vi "Daten zusammensammeln HovaCal.vi"(1 "KommLoopTimer":u32, 5 "Aktionen Daten abholen":T2, 7 "Aktion Unterbrechen":T1, 11 "error in (no error)":errorcluster caption="Fehler (Eingang, kein Fehler)") -> (4 "Anzeige aktualisieren":bool, 6 "Aktionen Daten abholen":T2, 8 "Aktion Unterbrechen out":T1, 10 "Zustand":string, 15 "error out":errorcluster caption="Fehler (Ausgang)")   [LabVIEW 2020, in "Linearisierung v2.lvlib"]
uses:
  Linearisierung v2.lvlib
  Daten abholen.ctl
  Gasteiler/Aktion unterbrechen.ctl
  Gasteiler/Aktion FGV Daten Abholung uebergebenctl.ctl
  Aktion FGV Stoerungen sammeln und auswerten.ctl
  Funktionstasten/Funktionstasten-Aktion.ctl
  Funktionstasten/Zustaende.ctl
  Seiten/FT-IR/Algebraic Modul/FGV Algebraic Aktionen.ctl
  Sprachverwaltung/FGV Aktion Tabelle zerlegen.ctl
  Seiten/FT-IR/FGV FT-IR Gasliste Aktionen.ctl
  Gasteiler/Aktionen FGV Gasteiler Daten.ctl
  Aktion Lin Daten aufarbeiten.ctl
  SpanEinstellungen/Aktion FGV GD Errors sammeln.ctl
  SpanEinstellungen/GD Info Cluster.ctl
  LIN ErrorCluster.ctl
  Funktionstasten/Funktionstasten.lvlib
  Allgemein/allgemeine Sub-VIs.lvlib
  Sprachverwaltung/Sprachverwaltung.lvlib
  Gasteiler/Gasteiler.lvlib
  Gasteiler/HovaCal/HovaCal.lvlib
  Gasteiler/HovaCal/Aktion_FGV_Betriebsdaten.ctl
  Gasteiler/HovaCal/Aktion_FGV_Kom.ctl
  Seiten/FT-IR/Algebraic Modul/Algebraic Modul.lvlib
  Seiten/FT-IR/FT-IR.lvlib
  Gasteiler/HovaCAL_Interface/Kommunikation/Kommunikation.lvlib
  Gasteiler/HovaCAL_Interface/HovaCAL_Interface.lvlib
  SpanEinstellungen/SpanEinstellungen.lvlib
  Gasteiler/HovaCAL_Interface/Helper/Helper.lvlib
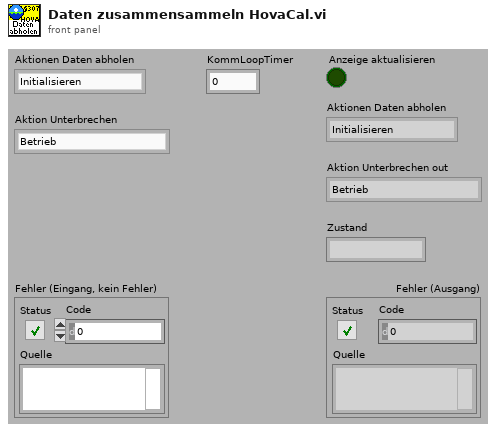
[diagram p1: front panel]
types:
  T1 = typedef "Linearisierung v2.lvlib/Gasteiler.lvlib/Aktion unterbrechen.ctl" = enum16{"Betrieb", "Unterbrechen", "Warten"}
  T2 = typedef "Linearisierung v2.lvlib/Daten abholen.ctl" = enum16{"Initialisieren", "Punkt aufschalten", "Warten", "Daten abholen", "Fertig", "Beenden", "Spülen", "Abbrechen"}
  T3 = typedef "Linearisierung v2.lvlib/Gasteiler.lvlib/Aktion FGV Daten Abholung uebergebenctl.ctl" = enum16{"lesen", "schreiben", "Anzeigebit löschen", "Status hinzufügen"}
  T4 = typedef "Linearisierung v2.lvlib/Aktion FGV Stoerungen sammeln und auswerten.ctl" = enum16{"init", "lesen", "error", "prüfen", "reset error", "abbrechen", "fortsetzen", "neustart", "Bedientasten reset"}
  T5 = typedef "Funktionstasten.lvlib/Zustaende.ctl" = enum16{"Standby", "Pause", "Eco", "Messen", "Kalibrieren", "Spülen Filter", "Spülen Leitung", "Umgebungsluft", "0-Gas", "Cal-Gas", "CG zu PNS", "-------------", "Init 1", "Init 2", "Init 3", "Init 4", "Messen vorbereiten", "Messen durchführen", "Exit"}
  T6 = typedef "Funktionstasten.lvlib/Funktionstasten-Aktion.ctl" = enum16{"Initialisieren", "Zustand setzen", "Taste gedrückt", "Fehler speichern", "Lesen", "Manuell", "Remote", "Bitparallel", "Samplepoint", "Zeit Prüfen", "reset Umschalten"}
  T7 = typedef "Linearisierung v2.lvlib/Aktion Lin Daten aufarbeiten.ctl" = enum16{"lesen", "Protkolldaten", "speichern", "laden", "EPA auswerten", "Tabelle schreiben", "Lin auswerten", "Tab init", "Stufentabelle", "EPA aktiviert", "Nachbehandlung laden", "Tabelle löschen", "Istwerte löschen", "Zeile löschen", "Zeile einfügen", "LIN aktiviert", "LIN/EPA aktiv laden", "EGAK Tab", "LIN übernehmen", "Tab init ohne Stufen"}
  T8 = typedef "Linearisierung v2.lvlib/Gasteiler.lvlib/Aktionen FGV Gasteiler Daten.ctl" = enum16{"lesen", "Gasteiler Daten", "Seriellen Param.", "MB-Endwert", "laden", "speichern", "Anforderung", "TCP", "Aufzeichnung Start"}
  T9 = typedef "FT-IR.lvlib/FGV FT-IR Gasliste Aktionen.ctl" = enum16{"lesen", "Gasliste FT-IR", "Gasliste ausgelesen", "laden", "speichern", "löschen"}
  T10 = typedef "Sprachverwaltung.lvlib/FGV Aktion Tabelle zerlegen.ctl" = enum16{"laden", "vereinzeln", "speichern"}
  T11 = typedef "FT-IR.lvlib/Algebraic Modul.lvlib/FGV Algebraic Aktionen.ctl" = enum16{"lesen", "laden", "speichern", "berechnen", "schreiben"}
  T12 = typedef "Linearisierung v2.lvlib/Gasteiler.lvlib/HovaCal.lvlib/Aktion_FGV_Kom.ctl" = enum16{"Initialisieren", "Betriebsparameter", "Gase", "Vaporizer", "Dynamische Werte", "Beenden", "Com ändern", "Gase init"}
  T13 = typedef "Linearisierung v2.lvlib/Gasteiler.lvlib/HovaCal.lvlib/Aktion_FGV_Betriebsdaten.ctl" = enum16{"Lesen", "Sollwerte schreiben", "Sollwerte lesen", "Gase schreiben", "Gase lesen", "Dynamische Werte", "GaseRef", "Gase aendern"}
  T14 = typedef "Linearisierung v2.lvlib/SpanEinstellungen.lvlib/GD Info Cluster.ctl" = cluster{"Wobei":string, "Status":string, "Errors":T15, "Empfangsdaten":string[], "Zeitstempel":string}
  T15 = typedef "Linearisierung v2.lvlib/LIN ErrorCluster.ctl" = cluster{"Störung Kommunikation":bool, "Pressure carrier gas":bool, "Pressure diluted gas":bool, "Outlet Pressure":bool, "SNOX before SAIR":bool, "Störung Gasteiler":bool}
  T16 = typedef "Linearisierung v2.lvlib/SpanEinstellungen.lvlib/Aktion FGV GD Errors sammeln.ctl" = enum16{"lesen", "init", "GD Infos sammeln", "Kalibrierinfos sammeln", "Test Data", "GD Infos selektiv sammeln"}
  T17 = typedef "Linearisierung v2.lvlib/Gasteiler.lvlib/HovaCal.lvlib/Betriebsdaten.ctl" = cluster{"Gesamtdurchfluss":dbl, "Eingangskonzentration \nTrägergas":dbl, "Eingangskonzentration\nKomponente 1":dbl, "Eingangskonzentration \nKomponente 2":dbl, "Ausgangskonzentration \nKomponente 1 ":dbl, "Ausgangskonzentration\nKomponente 2":dbl, "l/min -> ml/min":bool, "N2 %->ppm":bool, "Komp1 ppm->%":bool, "Komp2ppm->%":bool, "Sollkomp1ppm->%":bool, "Sollkomp2ppm->%":bool}
  T18 = typedef "Linearisierung v2.lvlib/Lin-Polynom Daten.ctl" = cluster{"Messgerät":string, "Kalibrator (Gasteiler)":string, "Bearbeiter/in":string, "Komponente":string, "Zeitstempel":timestamp, "F_max gefordert (%)":sgl, "F_max in %":sgl, "F_max in ppm":sgl, "Vorschlag Ordnung":i32, "Polynom OK":bool, "Polynomkoeff.":dbl[], "Prüfgas Konzentration":dbl, "Pfad EPA":string, "Pfad_LIN":string, "Gasnummer:":u8, "Komponentenauswahl":T19, "Verdünnungsgas":T21, "Zeitdauer Stufe":T22, "Anzahl Stufen":T22, "F_max in % EPA":sgl, "F_max in ppm EPA":sgl, "F_max in % LIN":sgl, "F_max in ppm LIN":sgl, "Punkte umkehren":bool, "EPA Optionsfeld":T23, "Autolin Hovacal":T24, "Spanfactors":sgl[], "Kalibrierauswahl":T25, "Conditions:":T26, "Gasflaschen Nr.:":string, "Bottle Accuracy":dbl, "Konfig Gasflasche":T27, "Gasflasche":T28, "HovaCAL Flow AutoLin":T29, "MFC Output":T30, "Gas Ablaufdatum":timestamp, "Lin Modus":T31, "zusätzliche Zeitdauer Erster Punkt":sgl, "Offsets":sgl[]}
  T19 = typedef "Linearisierung v2.lvlib/KomponentenArray.ctl" = cluster{"Komponente:":T20, "Konzentration":dbl}[]
  T20 = typedef "Auswahlfeld.ctl" = u16
  T21 = typedef "Linearisierung v2.lvlib/Gasteiler.lvlib/Prüfgas in.ctl" = u16
  T22 = typedef "Zahlen-Eingabefeld.ctl" = sgl
  T23 = typedef "Linearisierung v2.lvlib/EPA Optionsfeld.ctl" = enum32{"Istwert", "Rohwert", "Linearisierter Wert"}
  T24 = typedef "Linearisierung v2.lvlib/Gasteiler.lvlib/HovaCal.lvlib/AutoLin Hovacal.ctl" = enum32{"Keine Auswahl", "Optionsauswahl 1", "Optionsauswahl 2"}
  T25 = typedef "Linearisierung v2.lvlib/Kalibrieroption.ctl" = u16
  T26 = typedef "Linearisierung v2.lvlib/Linearity verification 1065-307.lvlib/Condition.ctl" = u16
  T27 = typedef "System Einstellungen V2.lvlib/Konfig Gasflasche.ctl" = bool
  T28 = typedef "System Einstellungen V2.lvlib/Gasflasche Auswahl.ctl" = u16
  T29 = typedef "Linearisierung v2.lvlib/Gasteiler.lvlib/HovaCAL_Interface.lvlib/Controls.lvlib/Flow Einstellung.ctl" = cluster{"HovaCAL Flow Input Cluster":dbl}
  T30 = typedef "Linearisierung v2.lvlib/Gasteiler.lvlib/HovaCAL_Interface.lvlib/Controls.lvlib/Pump state.ctl" = cluster{"Run":bool}
  T31 = typedef "CalGas Aufschaltung.lvlib/Lin Modus.ctl" = u16
  T32 = typedef "String - Ausgabefeld.ctl" = string
  T33 = typedef "Linearisierung v2.lvlib/Gasteiler.lvlib/Stufen Tabelle.ctl" = string[][]
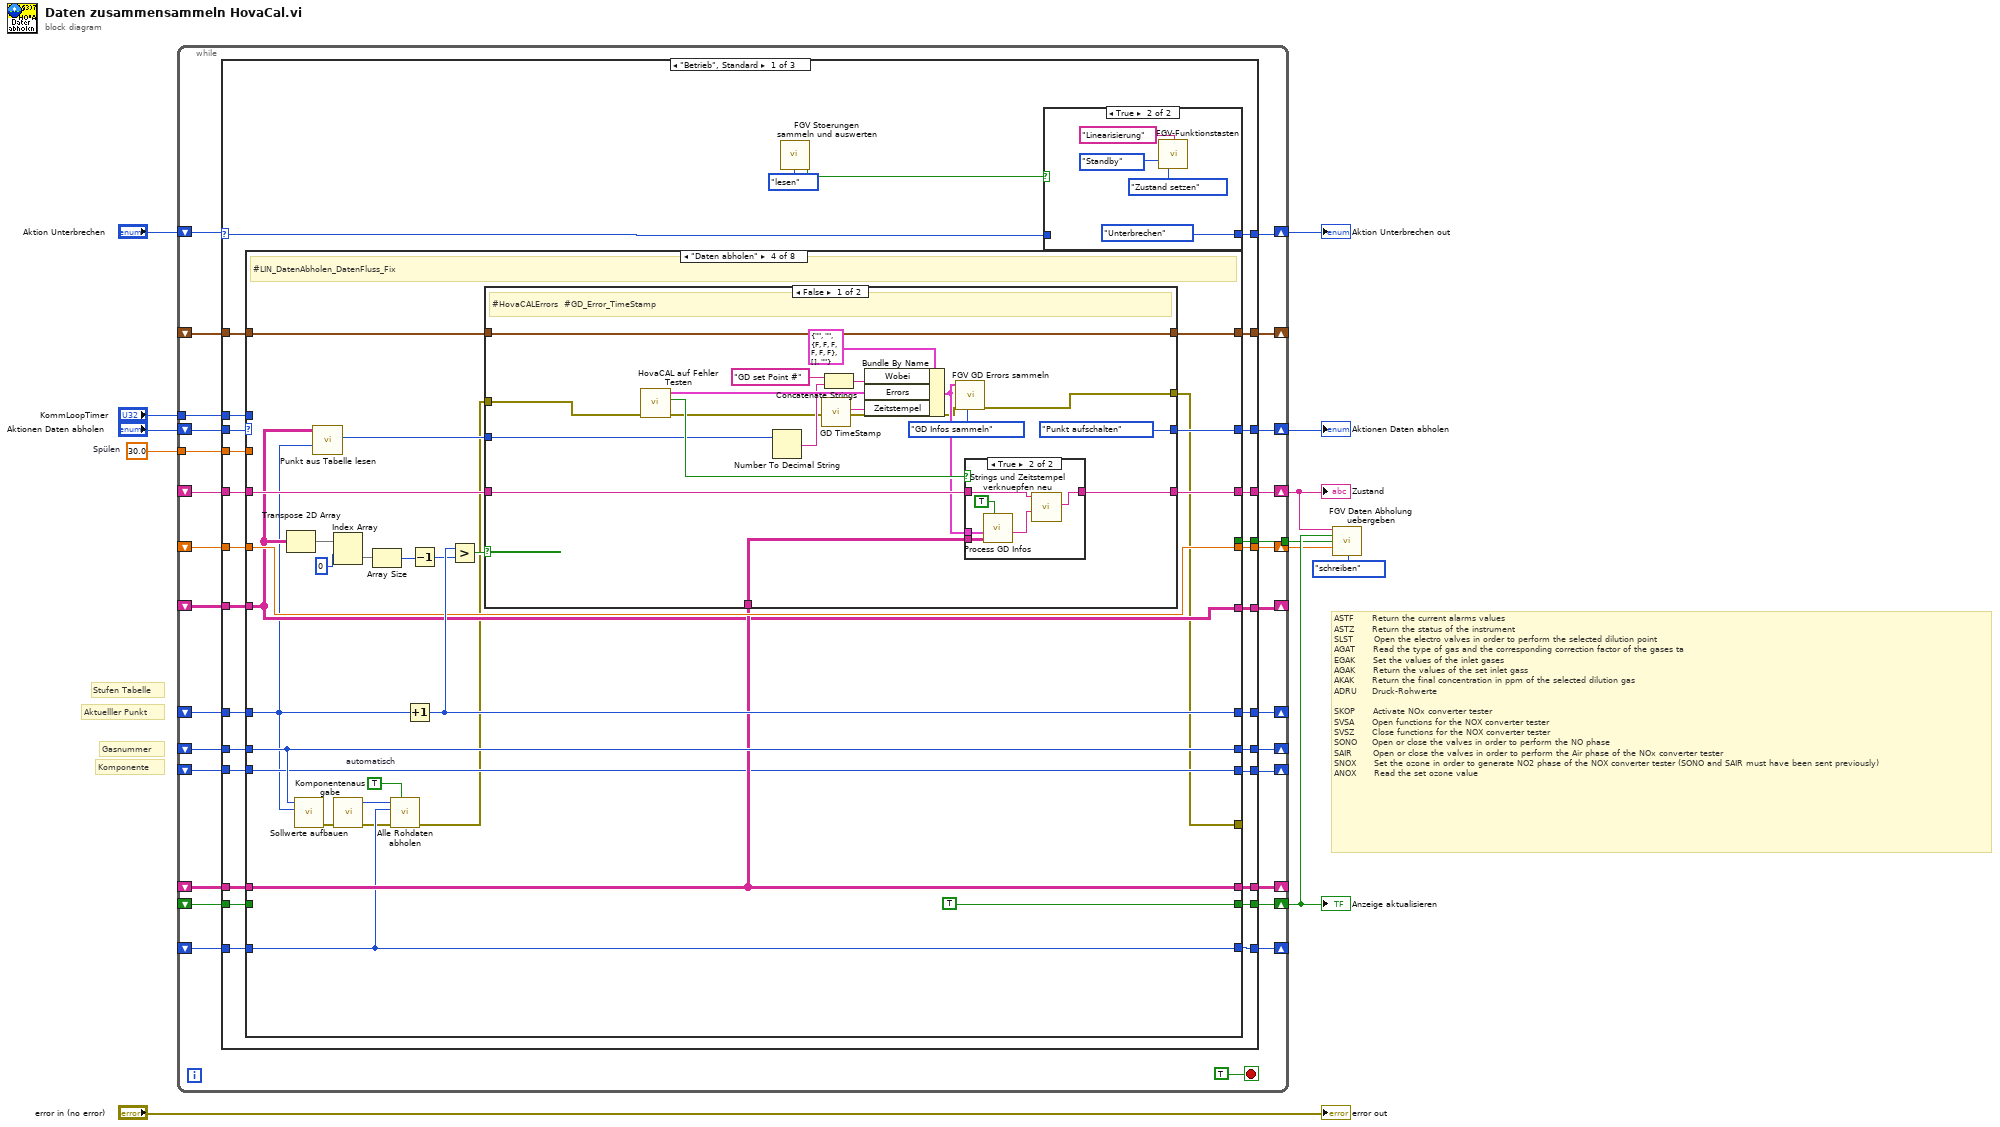
[diagram p0: block diagram]
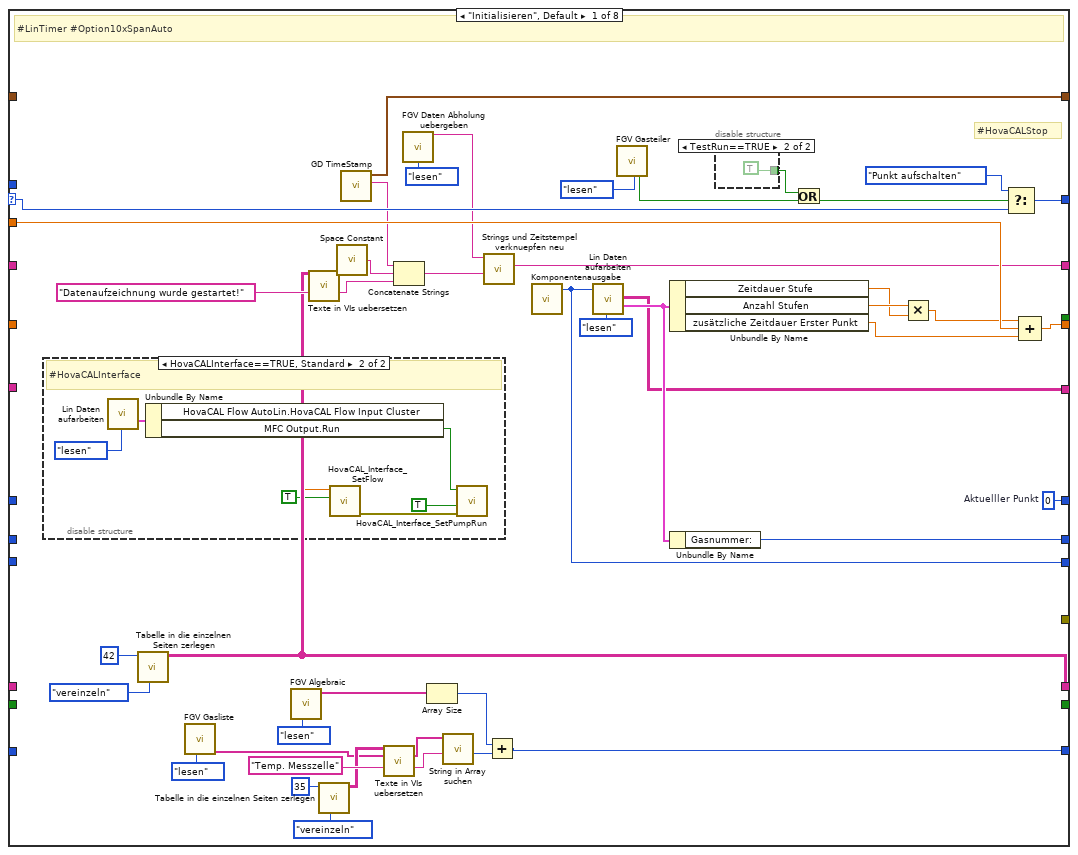
[diagram p3: hidden frame]
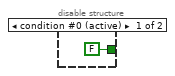
[diagram p4: hidden frame]
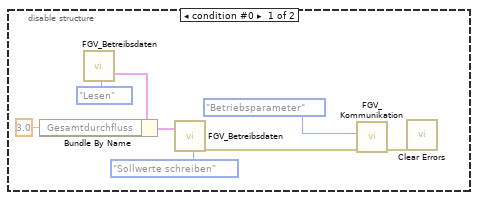
[diagram p5: hidden frame]
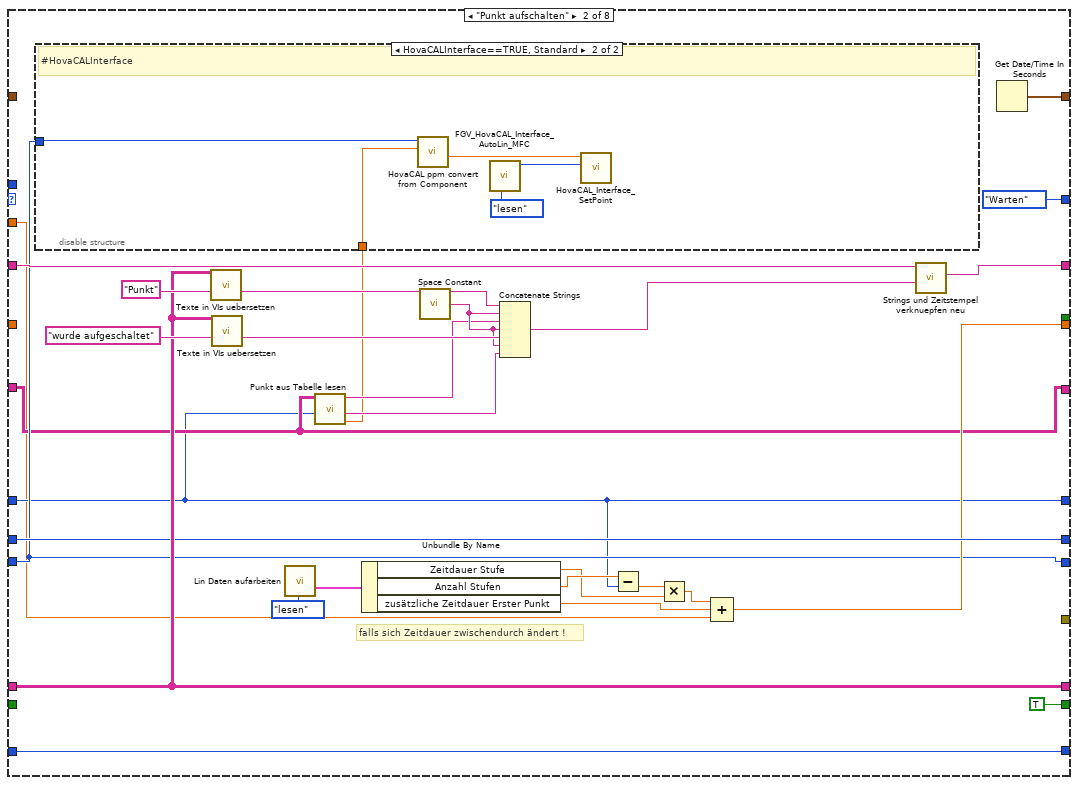
[diagram p6: hidden frame]
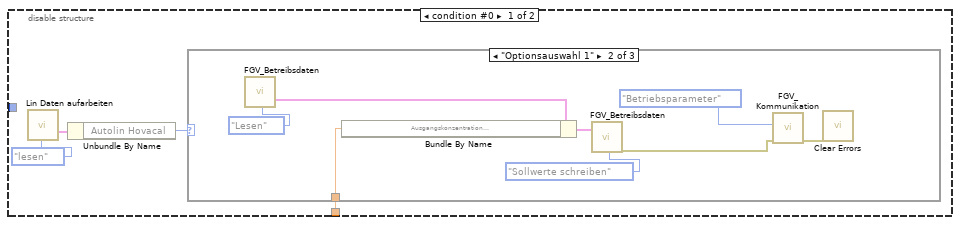
[diagram p7: hidden frame]
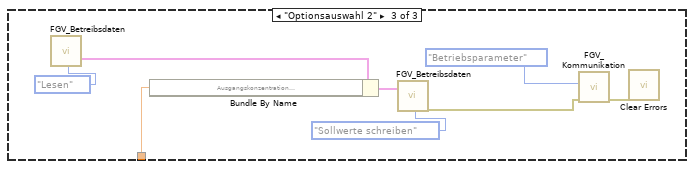
[diagram p9: hidden frame]
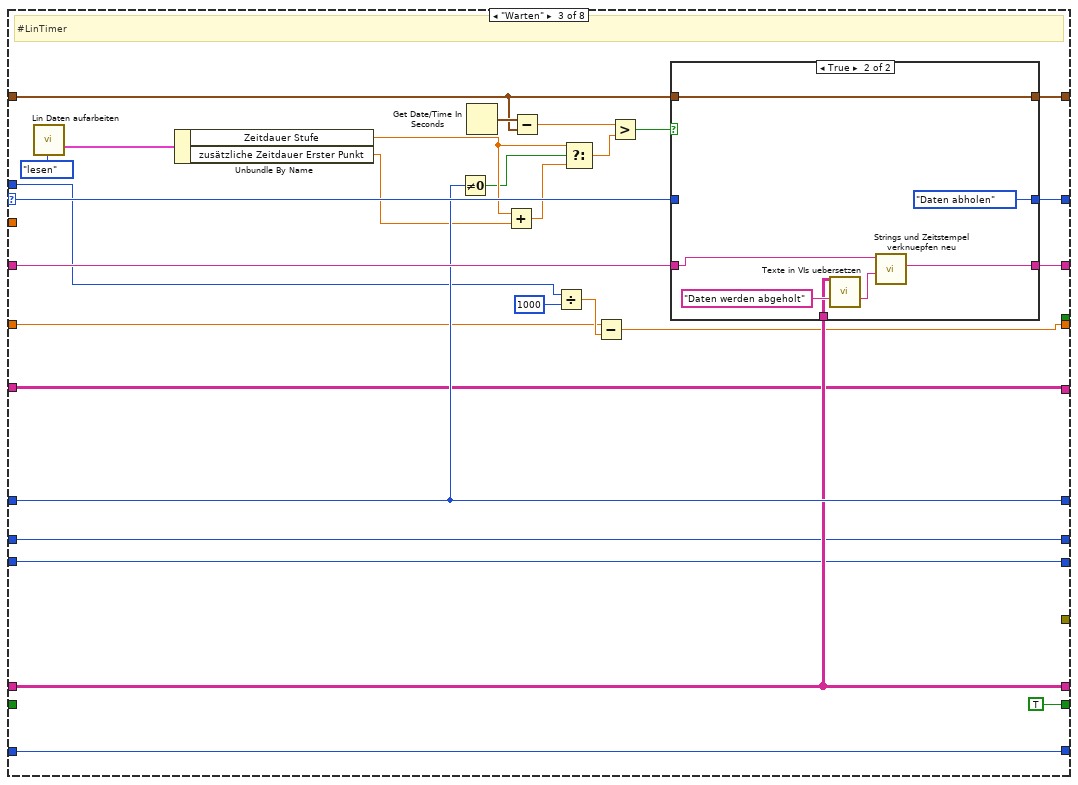
[diagram p10: hidden frame]
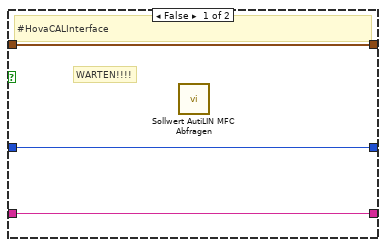
[diagram p11: hidden frame]
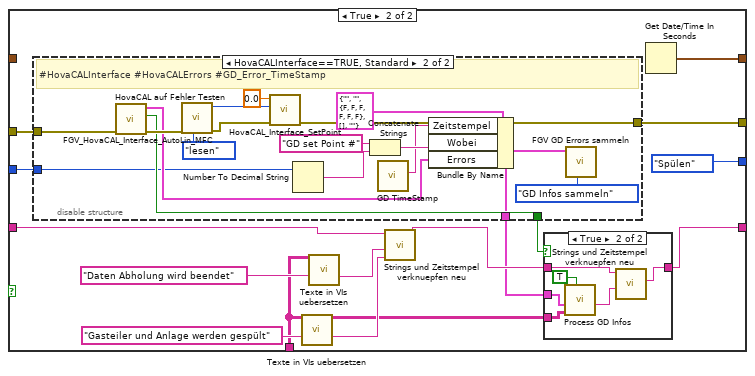
[diagram p13: hidden frame]
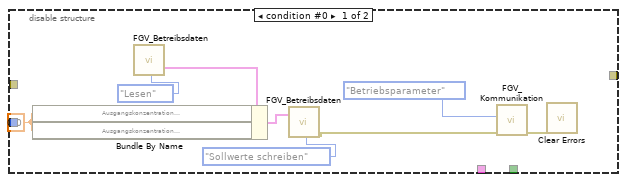
[diagram p15: hidden frame]
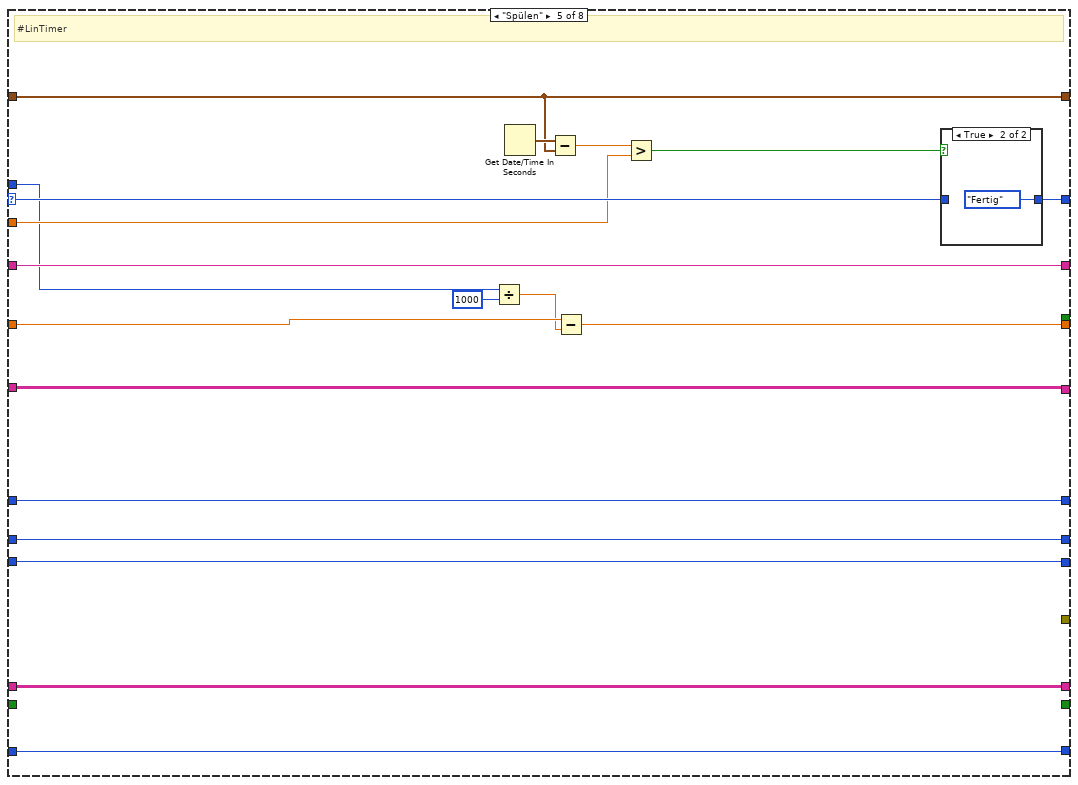
[diagram p16: hidden frame]
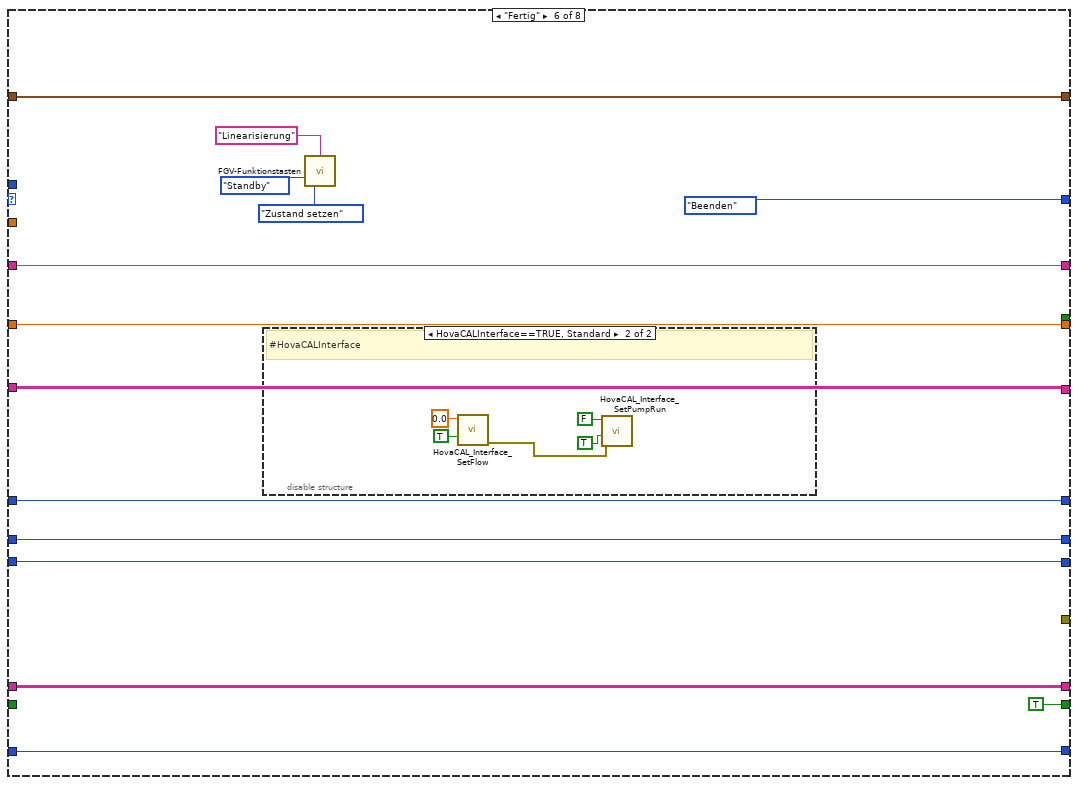
[diagram p18: hidden frame]
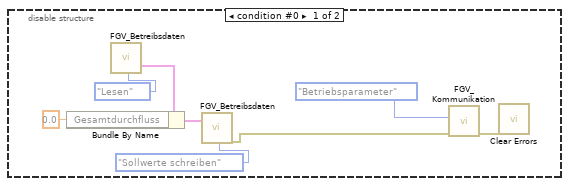
[diagram p19: hidden frame]
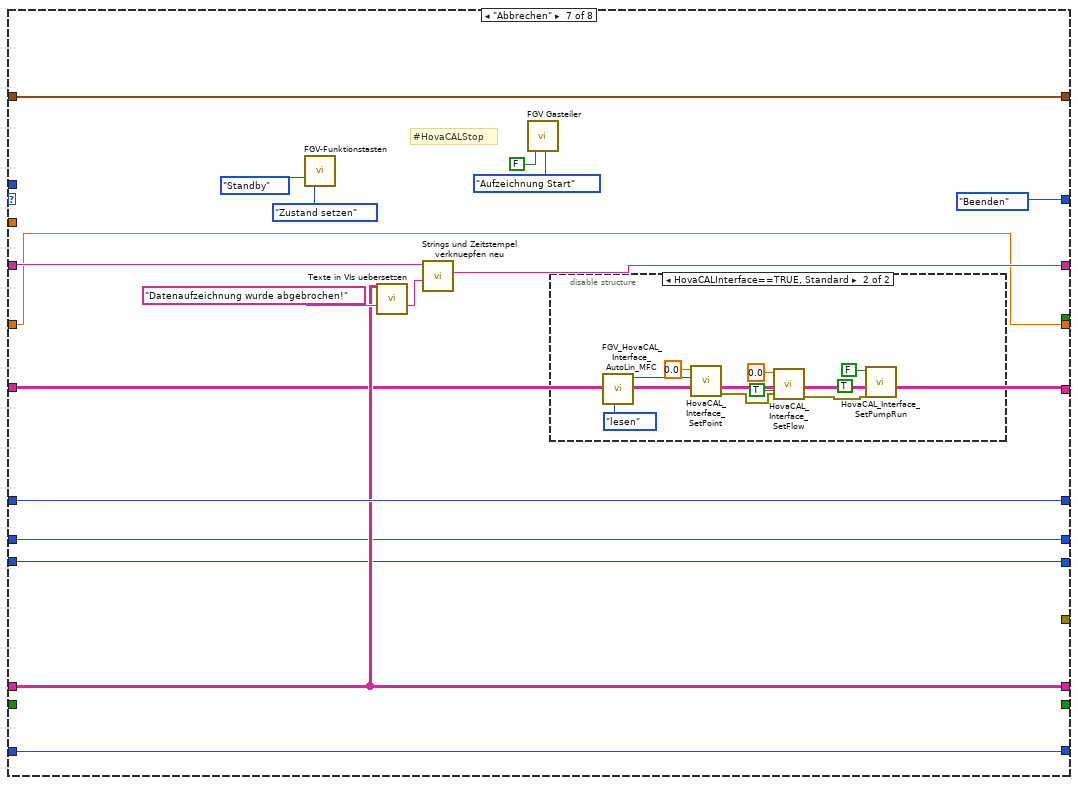
[diagram p20: hidden frame]
diagram:
  w5 = 30.0  # Spülen
  # "Komponente"
  # "Gasnummer"
  # "ASTF      Return the current alarms values\nASTZ      Return the status of the instrument \nSLST       Open the electro valves in order to perform the selected dilution point \nAGAT      Read the type of gas and the corresponding correction factor of the gases ta \nEGAK      Set the values of the inlet gases \nAGAK      Return the values of the set inlet gass \nAKAK      Return the final concentration in ppm of the selected dilution gas \nADRU     Druck-Rohwerte \n\nSKOP      Activate NOx converter tester \nSVSA      Open functions for the NOX converter tester \nSVSZ      Close functions for the NOX converter tester\nSONO     Open or close the valves in order to perform the NO phase\nSAIR       Open or close the valves in order to perform the Air phase of the NOx converter tester\nSNOX      Set the ozone in order to generate NO2 phase of the NOX converter tester (SONO and SAIR must have been sent previously)\nANOX      Read the set ozone value"
  # "Stufen Tabelle"
  # "Aktuelller Punkt"
  n1 = while {
    shift-right: [w38] -> _
    shift-left: _ -> [w39]
    shift-right: [w35] -> w10
    shift-left: _ -> [w34]
    shift-right: [w33] -> _
    shift-left: _ -> [w36]
    shift-right: [w30] -> _
    shift-left: _ -> [w31]
    shift-right: [w29] -> w9
    shift-left: _ -> [w28]
    shift-right: [w27] -> _
    shift-left: _ -> [w26]
    shift-right: [w37] -> w12
    shift-left: "Aktionen Daten abholen" -> [w40]
    tunnel: [w25] -> w8
    shift-right: [w24] -> _
    shift-left: _ -> [w23]
    shift-right: [w22] -> w6
    shift-left: _ -> [w21]
    tunnel: w5 -> [w20]
    tunnel: "KommLoopTimer" -> [w19]
    shift-right: [w17] -> w1
    shift-left: "Aktion Unterbrechen" -> [w18]
    shift-right: [w16] -> _
    shift-left: _ -> [w15]
    shift-right: [w14] -> _
    shift-left: _ -> [w13]
    stop <- TRUE stop-if-true
    n2 = case shown="\"Betrieb\", Standard" w18 {
      selector: w18 -> [w46 _ w460]
      tunnel: w40 -> [w69 w436 w454]
      tunnel: w39 -> [w68 w437 w470]
      tunnel: [w67 w437 w470] -> w38
      tunnel: [w66 w436 w458] -> w37
      tunnel: w36 -> [w65 w429 w467]
      tunnel: [w64 w432 w456] -> w35
      tunnel: w34 -> [w63 w433 w457]
      tunnel: [w62 w429 w467] -> w33
      tunnel: w31 -> [w61 w428 w455]
      tunnel: [w60 w428 w455] -> w30
      tunnel: [w59 w427 w469] -> w29
      tunnel: w28 -> [w58 w427 w469]
      tunnel: [w57 w426 w468] -> w27
      tunnel: w26 -> [w56 w426 w468]
      tunnel: [w55 _ _] -> w25
      tunnel: [w54 w430 w466] -> w24
      tunnel: w23 -> [w53 w430 w466]
      tunnel: [w52 w431 w465] -> w22
      tunnel: w21 -> [w51 w431 w465]
      tunnel: w20 -> [w50 _ _]
      tunnel: w19 -> [w49 _ _]
      tunnel: [w45 Aktion_unterbrechen."Warten" ("Aktion Unterbrechen") w459] -> w17
      tunnel: [w44 w425 w453] -> w16
      tunnel: w15 -> [w43 w425 w453]
      tunnel: [w42 w424 w452] -> w14
      tunnel: w13 -> [w41 w424 w452]
      frame "Betrieb", Default {
        n3 = case shown="\"Daten abholen\"" w69 {
          selector: w69 -> [w94 _ w209 _ w339 _ _ w421]
          tunnel: w68 -> [_ _ w210 w249 w341 w361 w391 w420]
          tunnel: [w75 w164 w211 w248 w341 w361 w391 w420] -> w67
          tunnel: [w97 Daten_abholen."Warten" ("Aktionen Daten abholen") w214 w254 w345 Daten_abholen."Beenden" ("Aktionen Daten abholen") Daten_abholen."Beenden" ("Aktionen Daten abholen") w421] -> w66
          tunnel: w63 -> [_ w163 w213 w251 w344 w359 w385 w422]
          tunnel: [w82 w162 w212 w250 w344 w359 w384 w422] -> w64
          tunnel: w65 -> [_ w140 w208 w234 w346 w362 w392 w423]
          tunnel: [w118 w140 w208 w253 w346 w362 w392 w423] -> w62
          tunnel: [w113 w156 w203 w243 w338 w356 w383 w419] -> w60
          tunnel: w61 -> [_ w156 w203 w243 w338 w356 w383 w419]
          tunnel: [_ TRUE TRUE TRUE _ TRUE _ TRUE] -> w59
          tunnel: w58 -> [_ _ _ _ _ _ _ _]
          tunnel: [w99 w154 w200 w233 w337 w355 w382 w418] -> w57
          tunnel: w56 -> [_ w154 w200 w233 w337 w355 w382 w418]
          tunnel: [_ _ _ _ _ _ _ TRUE] -> w55
          tunnel: [w77 w153 w199 w246 w336 w354 w381 w416] -> w54
          tunnel: w53 -> [_ w153 w199 w246 w336 w354 w381 w416]
          tunnel: [_ _ _ w228 _ _ _ _] -> _
          tunnel: [w91 w144 w193 w244 w333 w352 w378 w412] -> w52
          tunnel: w51 -> [_ _ w194 w244 w335 w352 w378 _]
          tunnel: w50 -> [w90 w136 _ _ w334 _ _ _]
          tunnel: w49 -> [_ _ w195 _ w332 _ _ _]
          tunnel: [w78 w142 w191 w242 w329 w350 w377 w411] -> w44
          tunnel: w43 -> [_ w142 w191 w242 w329 w350 w377 w411]
          tunnel: [w79 w141 w190 w236 w328 w349 w376 w410] -> w42
          tunnel: w41 -> [_ w141 w190 w236 w328 w349 w376 w410]
          frame "Initialisieren", Default {
            w118 = 0  # Aktuelller Punkt
            # "#HovaCALStop"
            # "#LinTimer #Option10xSpanAuto"
            n4 = disable-structure shown="HovaCALInterface==TRUE, Standard" {
              frame condition #0 {
                n5 = call "FGV_Betreibsdaten.vi"("Enum"=Aktion_FGV_Betriebsdaten."Lesen") -> ("Sollwert für Vergleich"=w126:T17)  [unwired: 11 in, 7 out]
                n6 = Bundle By Name(cluster=w126, "Gesamtdurchfluss"=3.0 ("Eingangskonzentration \nKomponente 2")) -> (w128:T17)
                n7 = call "FGV_Betreibsdaten.vi"("Sollwert schreiben"=w128, "Enum"=Aktion_FGV_Betriebsdaten."Sollwerte schreiben") -> ("error out"=w122:errorcluster)  [unwired: 10 in, 7 out]
                n8 = call "FGV_Kommunikation.vi"("error in"=w122, "Aktion"=Aktion_FGV_Kom."Betriebsparameter" ("Enum")) -> ("error out"=w121:errorcluster)  [unwired: 5 in, 4 out]
                n9 = call <vilib>:"Clear Errors.vi"("error in (no error)"=w121) -> ()  [unwired: 5 in, 2 out]
              }
              frame condition #1 (active) {
                # "#HovaCALInterface"
                n10 = call "Lin Daten aufarbeiten.vi"("Aktionen"=Aktion_Lin_Daten_aufarbeiten."lesen") -> ("Lin-Polynom"=w135:T18)  [unwired: 16 in, 10 out]
                n11 = Unbundle By Name(w135) -> ("HovaCAL Flow AutoLin.HovaCAL Flow Input Cluster"=w132:dbl, "MFC Output.Run"=w129:bool)
                n12 = call "HovaCAL_Interface_SetFlow.vi"("sofort"=TRUE, "total flow setpoint"=w132) -> ("error out"=w130:errorcluster)  [unwired: 9 in]
                n13 = call "HovaCAL_Interface_SetPumpRun.vi"("error in (no error)"=w130, "sofort"=TRUE, "run"=w129) -> ()  [unwired: 8 in, 1 out]
              }
            }
            n14 = call "Tabelle in die einzelnen Seiten zerlegen.vi"("Aktion"=FGV_Aktion_Tabelle_zerlegen."vereinzeln", "Index (Seite)"=42) -> ("Sprachliste"=w113:string[][])  [unwired: 7 in, 2 out]
            n15 = call "FGV Gasliste.vi"("Aktionen"=FGV_FT-IR_Gasliste_Aktionen."lesen") -> ("Aktuelle Gasliste gesamt"=w102:T32[])  [unwired: 8 in, 2 out]
            n16 = call "FGV Algebraic.vi"("Aktionen Algebraic"=FGV_Algebraic_Aktionen."lesen") -> ("Namen"=w104:string[])  [unwired: 6 in, 4 out]
            n17 = call "Texte in VIs uebersetzen.vi"("Sprachliste"=w113, "String zum Übersetzen"="Datenaufzeichnung wurde gestartet!" ("String 1 hinzufügen")) -> ("String zum Übersetzen"=w114:string)  [unwired: 9 in, 4 out]
            n18 = call "Tabelle in die einzelnen Seiten zerlegen.vi"("Aktion"=FGV_Aktion_Tabelle_zerlegen."vereinzeln", "Index (Seite)"=35) -> ("Sprachliste"=w105:string[][])  [unwired: 7 in, 2 out]
            n19 = call <vilib>:"Space Constant.vi"() -> ("String"=w117:string)
            n20 = call "GD TimeStamp.vi"() -> ("date/time string"=w76:string, "current time"=w75:timestamp)  [unwired: 10 in]
            n21 = call "Texte in VIs uebersetzen.vi"("Sprachliste"=w105, "String-Array zum Übersetzen"=w102, "String zum Übersetzen"="Temp. Messzelle" ("Neues Element/Teil-Array")) -> ("String-Array zum Übersetzen"=w101:string[], "String zum Übersetzen"=w107:string)  [unwired: 8 in, 3 out]
            n22 = Concatenate Strings(w76, w117, w114) -> (w83:string)
            n23 = call "FGV Daten Abholung uebergeben.vi"("Aktion"=Aktion_FGV_Daten_Abholung_uebergebenctl."lesen") -> ("Zustand"=w84:string)  [unwired: 10 in, 4 out]
            n24 = Array Size(array=w104) -> (size(s)=w109:i32)
            n25 = call "String in Array suchen.vi"("Nach String/Zeichen suchen (-)"=w107, "String-Array"=w101) -> ("Index"=w111:i32)  [unwired: 7 in, 2 out]
            n26 = call "Strings und Zeitstempel verknuepfen neu.vi"("String 1 hinzufügen"=w83, "Eingangs String"=w84) -> ("Verknüpfter String"=w82:string)  [unwired: 9 in]
            n27 = Add(x=w109, y=w111) -> (x+y=w99:i32)
            n28 = call "Komponentenausgabe.vi"() -> ("Gaskomponente"=w78:T20)  [unwired: 8 in, 3 out]
            n29 = call "Lin Daten aufarbeiten.vi"("Index (Seite)"=w78, "Aktionen"=Aktion_Lin_Daten_aufarbeiten."lesen") -> ("Stufen Tabelle"=w79:T33, "Lin-Polynom"=w87:T18)  [unwired: 15 in, 9 out]
            n30 = call "FGV Gasteiler.vi"("Aktionen"=Aktionen_FGV_Gasteiler_Daten."lesen") -> ("Aufzeichnung Start"=w96:bool)  [unwired: 11 in, 7 out]
            n31 = Unbundle By Name(w87) -> ("Zeitdauer Stufe"=w89:T22, "Anzahl Stufen"=w92:T22, "zusätzliche Zeitdauer Erster Punkt"=w86:sgl)
            n32 = Unbundle By Name(w87) -> ("Gasnummer:"=w77:u8)
            n33 = disable-structure shown="TestRun==TRUE" {
              disable-tunnel: [FALSE TRUE] -> w80
              frame condition #0 (active) {
              }
              frame condition #1 {
              }
            }
            n34 = Or(x=w80, y=w96) -> (x .or. y?=w81:bool)
            n35 = Multiply(x=w92, y=w89) -> (x*y=w88:T22)
            n36 = Select(t=Daten_abholen."Punkt aufschalten" ("Aktionen Daten abholen"), s=w81, f=w94) -> (s? t:f=w97:T2)
            n37 = Compound Arithmetic op=unknown(w88, w90, w86) -> (w91:dbl)
          }
          frame "Punkt aufschalten" {
            # "falls sich Zeitdauer zwischendurch ändert !"
            n38 = call "Texte in VIs uebersetzen.vi"("Sprachliste"=w156, "String zum Übersetzen"="Punkt" ("String 1 hinzufügen")) -> ("String zum Übersetzen"=w158:string)  [unwired: 9 in, 4 out]
            n39 = call "Texte in VIs uebersetzen.vi"("Sprachliste"=w156, "String zum Übersetzen"="wurde aufgeschaltet" ("String")) -> ("String zum Übersetzen"=w155:string)  [unwired: 9 in, 4 out]
            n40 = call "Lin Daten aufarbeiten.vi"("Aktionen"=Aktion_Lin_Daten_aufarbeiten."lesen") -> ("Lin-Polynom"=w146:T18)  [unwired: 16 in, 10 out]
            n41 = call "Punkt aus Tabelle lesen.vi"("Index"=w140, "Stufen Tabelle"=w141) -> (0:"Sollwert"=w137:sgl, 1:"Sollwert"=w138:string, "Punkt"=w139:string)  [unwired: 6 in, 1 out]
            n42 = disable-structure shown="HovaCALInterface==TRUE, Standard" {
              disable-tunnel: w137 -> [w165 w186]
              disable-tunnel: w142 -> [_ w187]
              frame condition #0 {
                n43 = call "Lin Daten aufarbeiten.vi"("Aktionen"=Aktion_Lin_Daten_aufarbeiten."lesen") -> ("Lin-Polynom"=w168:T18)  [unwired: 16 in, 10 out]
                n44 = Unbundle By Name(w168) -> ("Autolin Hovacal"=w166:T24)
                n45 = case shown="\"Optionsauswahl 1\"" w166 {
                  tunnel: w165 -> [_ w169 w177]
                  frame "Keine Auswahl", Default {
                  }
                  frame "Optionsauswahl 1" {
                    n46 = call "FGV_Betreibsdaten.vi"("Enum"=Aktion_FGV_Betriebsdaten."Lesen") -> ("Sollwert für Vergleich"=w175:T17)  [unwired: 11 in, 7 out]
                    n47 = Bundle By Name(cluster=w175, "Ausgangskonzentration \nKomponente 1"=w169) -> (w176:T17)
                    n48 = call "FGV_Betreibsdaten.vi"("Sollwert schreiben"=w176, "Enum"=Aktion_FGV_Betriebsdaten."Sollwerte schreiben") -> ("error out"=w170:errorcluster)  [unwired: 10 in, 7 out]
                    n49 = call "FGV_Kommunikation.vi"("error in"=w170, "Aktion"=Aktion_FGV_Kom."Betriebsparameter" ("Enum")) -> ("error out"=w171:errorcluster)  [unwired: 5 in, 4 out]
                    n50 = call <vilib>:"Clear Errors.vi"("error in (no error)"=w171) -> ()  [unwired: 5 in, 2 out]
                  }
                  frame "Optionsauswahl 2" {
                    n51 = call "FGV_Betreibsdaten.vi"("Enum"=Aktion_FGV_Betriebsdaten."Lesen") -> ("Sollwert für Vergleich"=w183:T17)  [unwired: 11 in, 7 out]
                    n52 = Bundle By Name(cluster=w183, "Ausgangskonzentration\nKomponente 2"=w177) -> (w184:T17)
                    n53 = call "FGV_Betreibsdaten.vi"("Sollwert schreiben"=w184, "Enum"=Aktion_FGV_Betriebsdaten."Sollwerte schreiben") -> ("error out"=w178:errorcluster)  [unwired: 10 in, 7 out]
                    n54 = call "FGV_Kommunikation.vi"("error in"=w178, "Aktion"=Aktion_FGV_Kom."Betriebsparameter" ("Enum")) -> ("error out"=w179:errorcluster)  [unwired: 5 in, 4 out]
                    n55 = call <vilib>:"Clear Errors.vi"("error in (no error)"=w179) -> ()  [unwired: 5 in, 2 out]
                  }
                }
              }
              frame condition #1 (active) {
                # "#HovaCALInterface"
                n56 = call "HovaCAL ppm convert from Component.vi"("Konzentration"=w186, "Gasnummer"=w187) -> ("Konzentration in ppm"=w185:dbl)  [unwired: 5 in, 4 out]
                n57 = call "FGV_HovaCAL_Interface_AutoLin_MFC.vi"("Aktion"=enum16{"lesen", "schreiben"}."lesen") -> ("AutoLin MFC out"=w188:u16)  [unwired: 7 in, 3 out]
                n58 = call "HovaCAL_Interface_SetPoint.vi"("AutoLin MFC Index"=w188, "Konzentration"=w185) -> ()  [unwired: 9 in, 1 out]
              }
            }
            n59 = Unbundle By Name(w146) -> ("Zeitdauer Stufe"=w148:T22, "Anzahl Stufen"=w149:T22, "zusätzliche Zeitdauer Erster Punkt"=w143:sgl)
            n60 = call <vilib>:"Space Constant.vi"() -> ("String"=w151:string)
            n61 = Concatenate Strings(w158, w151, w139, w151, w155, w151, w138) -> (w161:string)
            n62 = Subtract(x=w149, y=w140) -> (x-y=w145:T22)
            n63 = Multiply(x=w145, y=w148) -> (x*y=w147:T22)
            n64 = Compound Arithmetic op=unknown(w147, w143, w136) -> (w144:dbl)
            n65 = call "Strings und Zeitstempel verknuepfen neu.vi"("String 1 hinzufügen"=w161, "Eingangs String"=w163) -> ("Verknüpfter String"=w162:string)  [unwired: 9 in]
            n66 = Get Date/Time In Seconds() -> (seconds since 1Jan1904=w164:timestamp)
          }
          frame "Warten" {
            # "#LinTimer"
            n67 = call "Lin Daten aufarbeiten.vi"("Aktionen"=Aktion_Lin_Daten_aufarbeiten."lesen") -> ("Lin-Polynom"=w201:T18)  [unwired: 16 in, 10 out]
            n68 = Unbundle By Name(w201) -> ("Zeitdauer Stufe"=w207:T22, "zusätzliche Zeitdauer Erster Punkt"=w192:sgl)
            n69 = Not Equal To 0?(x=w208) -> (x != 0?=w205:bool)
            n70 = Get Date/Time In Seconds() -> (seconds since 1Jan1904=w217:timestamp)
            n71 = Add(x=w207, y=w192) -> (x+y=w206:T22)
            n72 = Subtract(x=w217, y=w210) -> (x-y=w216:dbl)
            n73 = Divide(x=w195, y=u32 1000) -> (x/y=w196:dbl)
            n74 = Select(t=w207, s=w205, f=w206) -> (s? t:f=w204:T22)
            n75 = Subtract(x=w194, y=w196) -> (x-y=w193:dbl)
            n76 = Greater?(x=w216, y=w204) -> (0:w215:bool)
            n77 = case shown="True" w215 {
              tunnel: [w220 Daten_abholen."Daten abholen" ("Aktionen Daten abholen")] -> w214
              tunnel: w213 -> [w219 w227]
              tunnel: [w219 w226] -> w212
              tunnel: [w218 w224] -> w211
              tunnel: w210 -> [w218 w224]
              tunnel: w209 -> [w220 _]
              tunnel: w203 -> [_ w221]
              frame False {
                # "WARTEN!!!!"
                # "#HovaCALInterface"
                n78 = call "Sollwert AutiLIN MFC Abfragen.vi"() -> ()  [unwired: 12 in]
              }
              frame True {
                n79 = call "Texte in VIs uebersetzen.vi"("Sprachliste"=w221, "String zum Übersetzen"="Daten werden abgeholt" ("String 1 hinzufügen")) -> ("String zum Übersetzen"=w222:string)  [unwired: 9 in, 4 out]
                n80 = call "Strings und Zeitstempel verknuepfen neu.vi"("String 1 hinzufügen"=w222, "Eingangs String"=w227) -> ("Verknüpfter String"=w226:string)  [unwired: 9 in]
              }
            }
          }
          frame "Daten abholen" {
            w245 = TRUE  # automatisch
            # "#LIN_DatenAbholen_DatenFluss_Fix"
            n81 = Transpose 2D Array(2D array=w236) -> (transposed array=w237:T33)
            n82 = call "Sollwerte aufbauen.vi"("Punkt"=w234, "Aktuelle Gasnummer"=w246) -> ("error out"=w231:errorcluster)  [unwired: 9 in]
            n83 = call "Punkt aus Tabelle lesen.vi"("Index"=w234, "Stufen Tabelle"=w236) -> ("Punkt"=w241:i32)  [unwired: 6 in, 3 out]
            n84 = Index Array(array=w237, index (row)=0 ("Index (Zeile)")) -> (element=w238:string[])  [unwired: 1 in]
            n85 = call "Komponentenausgabe.vi"("error in (no error)"=w231) -> ("error out"=w230:errorcluster, "Gaskomponente"=w232:T20)  [unwired: 7 in, 2 out]
            n86 = Array Size(array=w238) -> (size(s)=w239:i32)
            n87 = call "Alle Rohdaten abholen.vi"("automatisch"=w245, "error in (no error)"=w230, "Temp. Messzelle G-nr."=w233, "Gasindex"=w232) -> ("error out"=w229:errorcluster)  [unwired: 6 in, 1 out]
            n88 = Increment(x=w234) -> (x+1=w253:i32)
            n89 = Decrement(x=w239) -> (x-1=w235:i32)
            n90 = Greater?(x=w253, y=w235) -> (0:w252:bool)
            n91 = case shown="False" w252 {
              tunnel: [Daten_abholen."Punkt aufschalten" ("Aktionen Daten abholen") Daten_abholen."Spülen" ("Aktionen Daten abholen")] -> w254
              tunnel: w251 -> [w266 w294]
              tunnel: [w265 w285] -> w250
              tunnel: w249 -> [w271 _]
              tunnel: [w271 w293] -> w248
              tunnel: w243 -> [w264 w288]
              tunnel: w241 -> [w259 w282]
              tunnel: w229 -> [w257 w281]
              tunnel: [w255 w280] -> w228
              frame False {
                # "#HovaCALErrors  #GD_Error_TimeStamp"
                n92 = call "HovaCAL auf Fehler Testen.vi"("error in (no error)"=w257) -> ("error out"=w256:errorcluster, "Error"=w267:bool, "LNI Error Ausgangs-Cluster"=w263:T15)  [unwired: 8 in]
                n93 = Number To Decimal String(number=w259) -> (decimal integer string=w260:string)  [unwired: 1 in]
                n94 = call "GD TimeStamp.vi"() -> ("date/time string"=w258:string)  [unwired: 10 in, 1 out]
                n95 = Concatenate Strings("GD set Point #" ("Status"), w260) -> (w261:string)
                n96 = Bundle By Name(cluster=T14 {"Wobei"="", "Status"="", "Errors"={"Störung Kommunikation"=FALSE, "Pressure carrier gas"=FALSE, "Pressure diluted gas"=FALSE, "Outlet Pressure"=FALSE, "SNOX before SAIR"=FALSE, "Störung Gasteiler"=FALSE}, "Empfangsdaten"=[], "Zeitstempel"=""} ("GD Info-Cluster in"), "Wobei"=w261, "Errors"=w263, "Zeitstempel"=w258) -> (w262:T14)
                n97 = call "FGV GD Errors sammeln.vi"("Aktion"=Aktion_FGV_GD_Errors_sammeln."GD Infos sammeln", "error in (no error)"=w256, "GD Info-Cluster in"=w262) -> ("error out"=w255:errorcluster)  [unwired: 6 in, 2 out]
                n98 = case shown="True" w267 {
                  tunnel: w266 -> [w273 w279]
                  tunnel: [w273 w278] -> w265
                  tunnel: w264 -> [_ w277]
                  tunnel: w262 -> [_ w276]
                  frame False {
                  }
                  frame True {
                    n99 = call "Process GD Infos.vi"("show Status even if no Error"=TRUE, "Sprachliste"=w277, "GD Info-Cluster in"=w276) -> ("GD Infos"=w275:string)  [unwired: 6 in, 2 out]
                    n100 = call "Strings und Zeitstempel verknuepfen neu.vi"("String 1 hinzufügen"=w275, "Eingangs String"=w279) -> ("Verknüpfter String"=w278:string)  [unwired: 9 in]
                  }
                }
              }
              frame True {
                n101 = disable-structure shown="HovaCALInterface==TRUE, Standard" {
                  disable-tunnel: [_ w320] -> w287
                  disable-tunnel: [_ w318] -> w283
                  disable-tunnel: w282 -> [_ w316]
                  disable-tunnel: w281 -> [_ w313]
                  disable-tunnel: [_ w311] -> w280
                  frame condition #0 {
                    w309 = 0.0 ("Eingangskonzentration \nKomponente 2")
                    n102 = call "FGV_Betreibsdaten.vi"("Enum"=Aktion_FGV_Betriebsdaten."Lesen") -> ("Sollwert für Vergleich"=w308:T17)  [unwired: 11 in, 7 out]
                    n103 = Bundle By Name(cluster=w308, "Ausgangskonzentration \nKomponente 1"=w309, "Ausgangskonzentration\nKomponente 2"=w309) -> (w310:T17)
                    n104 = call "FGV_Betreibsdaten.vi"("Sollwert schreiben"=w310, "Enum"=Aktion_FGV_Betriebsdaten."Sollwerte schreiben") -> ("error out"=w303:errorcluster)  [unwired: 10 in, 7 out]
                    n105 = call "FGV_Kommunikation.vi"("error in"=w303, "Aktion"=Aktion_FGV_Kom."Betriebsparameter" ("Enum")) -> ("error out"=w304:errorcluster)  [unwired: 5 in, 4 out]
                    n106 = call <vilib>:"Clear Errors.vi"("error in (no error)"=w304) -> ()  [unwired: 5 in, 2 out]
                  }
                  frame condition #1 (active) {
                    # "#HovaCALInterface #HovaCALErrors #GD_Error_TimeStamp"
                    n107 = call "HovaCAL auf Fehler Testen.vi"("error in (no error)"=w313) -> ("error out"=w324:errorcluster, "Error"=w320:bool, "LNI Error Ausgangs-Cluster"=w319:T15)  [unwired: 8 in]
                    n108 = call "FGV_HovaCAL_Interface_AutoLin_MFC.vi"("Aktion"=enum16{"lesen", "schreiben"}."lesen", "error in (no error)"=w324) -> ("error out"=w312:errorcluster, "AutoLin MFC out"=w325:u16)  [unwired: 6 in, 2 out]
                    n109 = call "HovaCAL_Interface_SetPoint.vi"("error in (no error)"=w312, "AutoLin MFC Index"=w325, "Konzentration"=0.0) -> ("error out"=w311:errorcluster)  [unwired: 8 in]
                    n110 = Number To Decimal String(number=w316) -> (decimal integer string=w315:string)  [unwired: 1 in]
                    n111 = Concatenate Strings("GD set Point #" ("Status"), w315) -> (w317:string)
                    n112 = call "GD TimeStamp.vi"() -> ("date/time string"=w314:string)  [unwired: 10 in, 1 out]
                    n113 = Bundle By Name(cluster=T14 {"Wobei"="", "Status"="", "Errors"={"Störung Kommunikation"=FALSE, "Pressure carrier gas"=FALSE, "Pressure diluted gas"=FALSE, "Outlet Pressure"=FALSE, "SNOX before SAIR"=FALSE, "Störung Gasteiler"=FALSE}, "Empfangsdaten"=[], "Zeitstempel"=""} ("GD Info-Cluster in"), "Zeitstempel"=w314, "Wobei"=w317, "Errors"=w319) -> (w318:T14)
                    n114 = call "FGV GD Errors sammeln.vi"("Aktion"=Aktion_FGV_GD_Errors_sammeln."GD Infos sammeln", "GD Info-Cluster in"=w318) -> ()  [unwired: 7 in, 3 out]
                  }
                }
                n115 = call "Texte in VIs uebersetzen.vi"("Sprachliste"=w288, "String zum Übersetzen"="Gasteiler und Anlage werden gespült" ("String 2 hinzufügen")) -> ("Sprachliste out"=w284:string[][], "String zum Übersetzen"=w291:string)  [unwired: 9 in, 3 out]
                n116 = call "Texte in VIs uebersetzen.vi"("Sprachliste"=w288, "String zum Übersetzen"="Daten Abholung wird beendet" ("String 1 hinzufügen")) -> ("String zum Übersetzen"=w289:string)  [unwired: 9 in, 4 out]
                n117 = call "Strings und Zeitstempel verknuepfen neu.vi"("String 2 hinzufügen"=w291, "String 1 hinzufügen"=w289, "Eingangs String"=w294) -> ("Verknüpfter String"=w286:string)  [unwired: 8 in]
                n118 = case shown="True" w287 {
                  tunnel: w286 -> [w296 w302]
                  tunnel: [w296 w301] -> w285
                  tunnel: w284 -> [_ w299]
                  tunnel: w283 -> [_ w300]
                  frame False {
                  }
                  frame True {
                    n119 = call "Process GD Infos.vi"("show Status even if no Error"=TRUE, "Sprachliste"=w299, "GD Info-Cluster in"=w300) -> ("GD Infos"=w298:string)  [unwired: 6 in, 2 out]
                    n120 = call "Strings und Zeitstempel verknuepfen neu.vi"("String 1 hinzufügen"=w298, "Eingangs String"=w302) -> ("Verknüpfter String"=w301:string)  [unwired: 9 in]
                  }
                }
                n121 = Get Date/Time In Seconds() -> (seconds since 1Jan1904=w293:timestamp)
              }
            }
          }
          frame "Spülen" {
            # "#LinTimer"
            n122 = Divide(x=w332, y=u32 1000) -> (x/y=w330:dbl)
            n123 = Get Date/Time In Seconds() -> (seconds since 1Jan1904=w343:timestamp)
            n124 = Subtract(x=w343, y=w341) -> (x-y=w342:dbl)
            n125 = Subtract(x=w335, y=w330) -> (x-y=w333:dbl)
            n126 = Greater?(x=w342, y=w334) -> (0:w340:bool)
            n127 = case shown="True" w340 {
              tunnel: [w347 Daten_abholen."Fertig" ("Aktionen Daten abholen")] -> w345
              tunnel: w339 -> [w347 _]
              frame False {
              }
              frame True {
              }
            }
          }
          frame "Fertig" {
            n128 = disable-structure shown="HovaCALInterface==TRUE, Standard" {
              frame condition #0 {
                n129 = call "FGV_Betreibsdaten.vi"("Enum"=Aktion_FGV_Betriebsdaten."Lesen") -> ("Sollwert für Vergleich"=w368:T17)  [unwired: 11 in, 7 out]
                n130 = Bundle By Name(cluster=w368, "Gesamtdurchfluss"=0.0 ("Eingangskonzentration \nKomponente 2")) -> (w370:T17)
                n131 = call "FGV_Betreibsdaten.vi"("Sollwert schreiben"=w370, "Enum"=Aktion_FGV_Betriebsdaten."Sollwerte schreiben") -> ("error out"=w363:errorcluster)  [unwired: 10 in, 7 out]
                n132 = call "FGV_Kommunikation.vi"("error in"=w363, "Aktion"=Aktion_FGV_Kom."Betriebsparameter" ("Enum")) -> ("error out"=w364:errorcluster)  [unwired: 5 in, 4 out]
                n133 = call <vilib>:"Clear Errors.vi"("error in (no error)"=w364) -> ()  [unwired: 5 in, 2 out]
              }
              frame condition #1 (active) {
                # "#HovaCALInterface"
                n134 = call "HovaCAL_Interface_SetFlow.vi"("sofort"=TRUE, "total flow setpoint"=0.0) -> ("error out"=w371:errorcluster)  [unwired: 9 in]
                n135 = call "HovaCAL_Interface_SetPumpRun.vi"("error in (no error)"=w371, "sofort"=TRUE, "run"=FALSE) -> ()  [unwired: 8 in, 1 out]
              }
            }
            n136 = call "FGV-Funktionstasten.vi"("Herkunft"="Linearisierung", "Zustand"=Zustaende."Standby", "Aktion"=Funktionstasten-Aktion."Zustand setzen") -> ()  [unwired: 5 in, 8 out]
          }
          frame "Abbrechen" {
            # "#HovaCALStop"
            n137 = call "FGV-Funktionstasten.vi"("Zustand"=Zustaende."Standby", "Aktion"=Funktionstasten-Aktion."Zustand setzen") -> ()  [unwired: 6 in, 8 out]
            n138 = call "Texte in VIs uebersetzen.vi"("Sprachliste"=w383, "String zum Übersetzen"="Datenaufzeichnung wurde abgebrochen!" ("String 1 hinzufügen")) -> ("String zum Übersetzen"=w386:string)  [unwired: 9 in, 4 out]
            n139 = call "Strings und Zeitstempel verknuepfen neu.vi"("String 1 hinzufügen"=w386, "Eingangs String"=w385) -> ("Verknüpfter String"=w384:string)  [unwired: 9 in]
            n140 = call "FGV Gasteiler.vi"("Aufzeichnung Start"=FALSE, "Aktionen"=Aktionen_FGV_Gasteiler_Daten."Aufzeichnung Start") -> ()  [unwired: 10 in, 8 out]
            n141 = disable-structure shown="HovaCALInterface==TRUE, Standard" {
              frame condition #0 {
                # "#HovaCALInterface"
                n142 = call "FGV_Betreibsdaten.vi"("Enum"=Aktion_FGV_Betriebsdaten."Lesen") -> ("Sollwert für Vergleich"=w398:T17)  [unwired: 11 in, 7 out]
                n143 = Bundle By Name(cluster=w398, "Gesamtdurchfluss"=0.0 ("Eingangskonzentration \nKomponente 2")) -> (w400:T17)
                n144 = call "FGV_Betreibsdaten.vi"("Sollwert schreiben"=w400, "Enum"=Aktion_FGV_Betriebsdaten."Sollwerte schreiben") -> ("error out"=w393:errorcluster)  [unwired: 10 in, 7 out]
                n145 = call "FGV_Kommunikation.vi"("error in"=w393, "Aktion"=Aktion_FGV_Kom."Betriebsparameter" ("Enum")) -> ("error out"=w394:errorcluster)  [unwired: 5 in, 4 out]
                n146 = call <vilib>:"Clear Errors.vi"("error in (no error)"=w394) -> ()  [unwired: 5 in, 2 out]
              }
              frame condition #1 (active) {
                n147 = call "FGV_HovaCAL_Interface_AutoLin_MFC.vi"("Aktion"=enum16{"lesen", "schreiben"}."lesen") -> ("AutoLin MFC out"=w403:u16)  [unwired: 7 in, 3 out]
                n148 = call "HovaCAL_Interface_SetPoint.vi"("AutoLin MFC Index"=w403, "Konzentration"=0.0) -> ("error out"=w401:errorcluster)  [unwired: 9 in]
                n149 = call "HovaCAL_Interface_SetFlow.vi"("error in (no error)"=w401, "sofort"=TRUE, "total flow setpoint"=0.0) -> ("error out"=w405:errorcluster)  [unwired: 8 in]
                n150 = call "HovaCAL_Interface_SetPumpRun.vi"("error in (no error)"=w405, "sofort"=TRUE, "run"=FALSE) -> ()  [unwired: 8 in, 1 out]
              }
            }
          }
          frame "Beenden" {
            w412 = sgl 0.0  # Restlaufzeit
            # "#HovaCALStop"
            # "#LinTimer"
            n151 = call "FGV Gasteiler.vi"("Aufzeichnung Start"=FALSE, "Aktionen"=Aktionen_FGV_Gasteiler_Daten."Aufzeichnung Start") -> ()  [unwired: 10 in, 8 out]
          }
        }
        n152 = call "FGV Stoerungen sammeln und auswerten.vi"("Aktion"=Aktion_FGV_Stoerungen_sammeln_und_auswerten."lesen") -> ("Error"=w47:bool)  [unwired: 12 in, 6 out]
        n153 = case shown="True" w47 {
          tunnel: [w70 Aktion_unterbrechen."Unterbrechen" ("Aktion Unterbrechen")] -> w45
          tunnel: w46 -> [w70 _]
          frame False {
          }
          frame True {
            n154 = call "FGV-Funktionstasten.vi"("Herkunft"="Linearisierung", "Zustand"=Zustaende."Standby", "Aktion"=Funktionstasten-Aktion."Zustand setzen") -> ()  [unwired: 5 in, 8 out]
          }
        }
      }
      frame "Unterbrechen" {
        n155 = disable-structure shown="HovaCALInterface==TRUE, Standard" {
          frame condition #0 {
            n156 = call "FGV_Betreibsdaten.vi"("Enum"=Aktion_FGV_Betriebsdaten."Lesen") -> ("Sollwert für Vergleich"=w444:T17)  [unwired: 11 in, 7 out]
            n157 = Bundle By Name(cluster=w444, "Gesamtdurchfluss"=0.0 ("Eingangskonzentration \nKomponente 2")) -> (w446:T17)
            n158 = call "FGV_Betreibsdaten.vi"("Sollwert schreiben"=w446, "Enum"=Aktion_FGV_Betriebsdaten."Sollwerte schreiben") -> ("error out"=w439:errorcluster)  [unwired: 10 in, 7 out]
            n159 = call "FGV_Kommunikation.vi"("error in"=w439, "Aktion"=Aktion_FGV_Kom."Betriebsparameter" ("Enum")) -> ("error out"=w440:errorcluster)  [unwired: 5 in, 4 out]
            n160 = call <vilib>:"Clear Errors.vi"("error in (no error)"=w440) -> ()  [unwired: 5 in, 2 out]
          }
          frame condition #1 (active) {
            # "#HovaCALInterface"
            n161 = call "HovaCAL_Interface_SetFlow.vi"("sofort"=TRUE, "total flow setpoint"=0.0) -> ("error out"=w447:errorcluster)  [unwired: 9 in]
            n162 = call "HovaCAL_Interface_SetPumpRun.vi"("error in (no error)"=w447, "sofort"=TRUE, "run"=FALSE) -> ()  [unwired: 8 in, 1 out]
          }
        }
        n163 = call "Texte in VIs uebersetzen.vi"("Sprachliste"=w428, "String zum Übersetzen"="Datenaufzeichnung wurde aufgrund eines Fehlers angehalten." ("String 1 hinzufügen")) -> ("String zum Übersetzen"=w435:string)  [unwired: 9 in, 4 out]
        n164 = call "Strings und Zeitstempel verknuepfen neu.vi"("String 1 hinzufügen"=w435, "Eingangs String"=w433) -> ("Verknüpfter String"=w432:string)  [unwired: 9 in]
      }
      frame "Warten" {
        n165 = call "FGV Stoerungen sammeln und auswerten.vi"("Aktion"=Aktion_FGV_Stoerungen_sammeln_und_auswerten."lesen") -> ("Neustart"=w462:bool, "Abbrechen"=w463:bool, "Fortsetzen"=w461:bool)  [unwired: 12 in, 4 out]
        n166 = case shown="False" w463 {
          tunnel: [Daten_abholen."Abbrechen" ("Aktionen Daten abholen") w483] -> w458
          tunnel: w462 -> [_ w482]
          tunnel: w461 -> [_ w481]
          tunnel: w454 -> [_ w480]
          tunnel: [Aktion_unterbrechen."Betrieb" ("Aktion Unterbrechen") w479] -> w459
          tunnel: w460 -> [_ w478]
          tunnel: w457 -> [w471 w477]
          tunnel: [w471 w476] -> w456
          tunnel: w455 -> [_ w475]
          frame True {
            # "Abbrechen"
            n167 = call "FGV Stoerungen sammeln und auswerten.vi"("Aktion"=Aktion_FGV_Stoerungen_sammeln_und_auswerten."Bedientasten reset") -> ()  [unwired: 12 in, 7 out]
          }
          frame False {
            # "Abbrechen"
            n168 = case shown="True" w482 {
              tunnel: [Daten_abholen."Initialisieren" ("Aktionen Daten abholen") w514] -> w483
              tunnel: w481 -> [_ w513]
              tunnel: w480 -> [_ w510]
              tunnel: [Aktion_unterbrechen."Betrieb" ("Aktion Unterbrechen") w512] -> w479
              tunnel: w478 -> [_ w511]
              tunnel: w477 -> [w494 w509]
              tunnel: [w493 w508] -> w476
              tunnel: w475 -> [w492 w507]
              tunnel: [w484 _] -> _
              frame True {
                # "Neustart"
                n169 = call "Lin Daten aufarbeiten.vi"("Aktionen"=Aktion_Lin_Daten_aufarbeiten."lesen") -> ("Lin-Polynom"=w491:T18)  [unwired: 16 in, 10 out]
                n170 = Unbundle By Name(w491) -> ("Lin Modus"=w489:T31)
                n171 = case shown="1, Standard" w489 {
                  tunnel: [Zustaende."Cal-Gas" ("Zustand") Zustaende."Messen" ("Zustand") Zustaende."CG zu PNS" ("Zustand")] -> w488
                  frame 1, Default {
                    # "Cal Gas to Samplepoint"
                  }
                  frame 2 {
                    # "Measure"
                  }
                  frame 0 {
                    # "Cal Gas to PNS"
                  }
                }
                n172 = call "FGV-Funktionstasten.vi"("Herkunft"="Linearisierung", "Zustand"=w488, "Aktion"=Funktionstasten-Aktion."Zustand setzen") -> ("Fehler steht an"=w486:bool)  [unwired: 5 in, 7 out]
                n173 = disable-structure shown="Deaktiviert" {
                  disable-tunnel: [w502 _] -> w485
                  disable-tunnel: w486 -> [w501 _]
                  frame Disabled {
                    # "UNKLAR !"
                    n174 = call "warten.vi"("Datenfluss"=w501, "Zu wartende ms"=u32 3000) -> ("error out"=w502:errorcluster)  [unwired: 8 in, 1 out]
                  }
                  frame Enabled {
                  }
                }
                n175 = call "Texte in VIs uebersetzen.vi"("Sprachliste"=w492, "String zum Übersetzen"="Datenaufzeichnung wird neu gestartet." ("String 1 hinzufügen")) -> ("String zum Übersetzen"=w495:string)  [unwired: 9 in, 4 out]
                n176 = call "Strings und Zeitstempel verknuepfen neu.vi"("String 1 hinzufügen"=w495, "Eingangs String"=w494) -> ("Verknüpfter String"=w493:string)  [unwired: 9 in]
                n177 = call "FGV Stoerungen sammeln und auswerten.vi"("error in (no error)"=w485, "Aktion"=Aktion_FGV_Stoerungen_sammeln_und_auswerten."Bedientasten reset") -> ("error out"=w484:errorcluster)  [unwired: 11 in, 6 out]
              }
              frame False {
                # "Neustart"
                n178 = case shown="True" w513 {
                  tunnel: [w517 w518] -> w514
                  tunnel: w510 -> [w517 w518]
                  tunnel: [w516 Aktion_unterbrechen."Betrieb" ("Aktion Unterbrechen")] -> w512
                  tunnel: w511 -> [w516 _]
                  tunnel: w509 -> [w515 w530]
                  tunnel: [w515 w529] -> w508
                  tunnel: w507 -> [_ w528]
                  tunnel: [_ w519] -> _
                  frame False {
                    # "Fortsetzen"
                  }
                  frame True {
                    # "bleibt in Punkt aufschalten \noder Spülen !"
                    # "Fortsetzen"
                    n179 = call "Lin Daten aufarbeiten.vi"("Aktionen"=Aktion_Lin_Daten_aufarbeiten."lesen") -> ("Lin-Polynom"=w527:T18)  [unwired: 16 in, 10 out]
                    n180 = Unbundle By Name(w527) -> ("Lin Modus"=w525:T31)
                    n181 = case shown="1, Standard" w525 {
                      tunnel: [Zustaende."Cal-Gas" ("Zustand") Zustaende."Cal-Gas" ("Zustand") Zustaende."Messen" ("Zustand") Zustaende."Cal-Gas" ("Zustand")] -> w524
                      frame 0 {
                        # "Cal Gas to PNS"
                      }
                      frame 1, Default {
                        # "Cal Gas to Samplepoint"
                      }
                      frame 2 {
                        # "Measure"
                      }
                      frame 3 {
                        # "Gasdivider"
                      }
                    }
                    n182 = call "FGV-Funktionstasten.vi"("Herkunft"="Linearisierung", "Zustand"=w524, "Aktion"=Funktionstasten-Aktion."Zustand setzen") -> ("Fehler steht an"=w522:bool)  [unwired: 5 in, 7 out]
                    n183 = call "Texte in VIs uebersetzen.vi"("Sprachliste"=w528, "String zum Übersetzen"="Datenaufzeichnung wird fortgesetzt." ("String 1 hinzufügen")) -> ("String zum Übersetzen"=w531:string)  [unwired: 9 in, 4 out]
                    n184 = disable-structure shown="Deaktiviert" {
                      disable-tunnel: [w537 _] -> w521
                      disable-tunnel: w522 -> [w536 _]
                      frame Disabled {
                        # "UNKLAR !"
                        n185 = call "warten.vi"("Datenfluss"=w536, "Zu wartende ms"=u32 3000) -> ("error out"=w537:errorcluster)  [unwired: 8 in, 1 out]
                      }
                      frame Enabled {
                      }
                    }
                    n186 = disable-structure shown="HovaCALInterface==TRUE, Standard" {
                      disable-tunnel: w521 -> [_ w548]
                      disable-tunnel: [_ w547] -> w520
                      frame condition #0 {
                        n187 = call "FGV_Betreibsdaten.vi"("Enum"=Aktion_FGV_Betriebsdaten."Lesen") -> ("Sollwert für Vergleich"=w544:T17)  [unwired: 11 in, 7 out]
                        n188 = Bundle By Name(cluster=w544, "Gesamtdurchfluss"=3.0 ("Eingangskonzentration \nKomponente 2")) -> (w546:T17)
                        n189 = call "FGV_Betreibsdaten.vi"("Sollwert schreiben"=w546, "Enum"=Aktion_FGV_Betriebsdaten."Sollwerte schreiben") -> ("error out"=w540:errorcluster)  [unwired: 10 in, 7 out]
                        n190 = call "FGV_Kommunikation.vi"("error in"=w540, "Aktion"=Aktion_FGV_Kom."Betriebsparameter" ("Enum")) -> ("error out"=w539:errorcluster)  [unwired: 5 in, 4 out]
                        n191 = call <vilib>:"Clear Errors.vi"("error in (no error)"=w539) -> ()  [unwired: 5 in, 2 out]
                      }
                      frame condition #1 (active) {
                        # "#HovaCALInterface"
                        n192 = call "Lin Daten aufarbeiten.vi"("error in (no error)"=w548, "Aktionen"=Aktion_Lin_Daten_aufarbeiten."lesen") -> ("Lin-Polynom"=w555:T18)  [unwired: 15 in, 10 out]
                        n193 = Unbundle By Name(w555) -> ("HovaCAL Flow AutoLin.HovaCAL Flow Input Cluster"=w552:dbl, "MFC Output.Run"=w549:bool)
                        n194 = call "HovaCAL_Interface_SetFlow.vi"("sofort"=TRUE, "total flow setpoint"=w552) -> ("error out"=w550:errorcluster)  [unwired: 9 in]
                        n195 = call "HovaCAL_Interface_SetPumpRun.vi"("error in (no error)"=w550, "sofort"=TRUE, "run"=w549) -> ("error out"=w547:errorcluster)  [unwired: 8 in]
                      }
                    }
                    n196 = call "Strings und Zeitstempel verknuepfen neu.vi"("String 1 hinzufügen"=w531, "Eingangs String"=w530) -> ("Verknüpfter String"=w529:string)  [unwired: 9 in]
                    n197 = call "FGV Stoerungen sammeln und auswerten.vi"("error in (no error)"=w520, "Aktion"=Aktion_FGV_Stoerungen_sammeln_und_auswerten."Bedientasten reset") -> ("error out"=w519:errorcluster)  [unwired: 11 in, 6 out]
                  }
                }
              }
            }
          }
        }
      }
    }
  }
  "Zustand" <- w10
  "Aktionen Daten abholen" <- w12
  "Anzeige aktualisieren" <- w9
  "Aktion Unterbrechen out" <- w1
  n198 = call "FGV Daten Abholung uebergeben.vi"("Zustand"=w10, "Anzeige aktualisieren"=w9, "Beendet"=w8, "Restlaufzeit"=w6, "Aktion"=Aktion_FGV_Daten_Abholung_uebergebenctl."schreiben") -> ()  [unwired: 6 in, 5 out]
  "error out" <- "error in (no error)"
